vi "brightness.vi"(2 "brightness":dbl, 3 "Colocr_in":u32(colorbox)) -> (1 "Color_out":u32(colorbox))   [LabVIEW 2011]
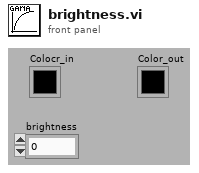
[diagram p1: front panel]
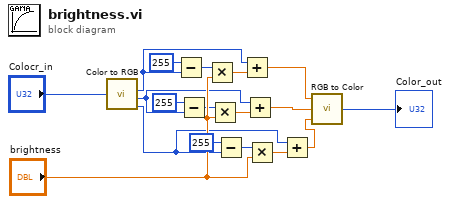
[diagram p0: block diagram]
diagram:
  n1 = call <vilib>:"Color to RGB.vi"("Color"="Colocr_in") -> ("R"=w5:u8, "G"=w9:u8, "B"=w16:u8)  [unwired: 1 out]
  n2 = Subtract(x=u32 255 ("y"), y=w5) -> (x-y=w3:u32)
  n3 = Subtract(x=u32 255 ("y"), y=w9) -> (x-y=w7:u32)
  n4 = Multiply(x=w3, y="brightness") -> (x*y=w4:dbl)
  n5 = Multiply(x=w7, y="brightness") -> (x*y=w6:dbl)
  n6 = Subtract(x=u32 255 ("y"), y=w16) -> (x-y=w14:u32)
  n7 = Add(x=w5, y=w4) -> (x+y=w10:dbl)
  n8 = Add(x=w9, y=w6) -> (x+y=w11:dbl)
  n9 = Multiply(x=w14, y="brightness") -> (x*y=w13:dbl)
  n10 = Add(x=w16, y=w13) -> (x+y=w17:dbl)
  n11 = call <vilib>:"RGB to Color.vi"("B"=w17, "G"=w11, "R"=w10) -> ("Color"=→"Color_out":u32)
